vi "Read_I2C_Data.vi"(8 "Error_In":errorcluster, 11 "I2C_In":refnum<class "I2C.lvclass">) -> (0 "Error_Out":errorcluster, 2 "Convertor_Data":T1={"Vmin"=0.0, "Vmax"=1.0, "Input"="", "Off_Set (uS)"=0.0, "T_HD_STA (uS)"=0.0, "Sample_Per_Us"=0.0, "T_HD_DAT (uS)"=0.0, "T_SU_DAT (uS)"=0.0, "Frequency (kHz)"=0.0, "T_SU_STO"=0.0, "T_Off (uS)"=0.0, "T_On (uS)"=0.0, "T_BUF"=0.0, "Target_Address"=0, "Selected_Register_Address"=0, "Byte_Array"=[], "Target_Name"="", "Register_Name"=[], "Register_Address"=[], "Target_Type"=0, "Register_Data"=[]} {"Target_Type" items=["10 Bit Address", "7 Bit Address"]; "Selected_Register_Address" format="%x"; "Target_Address" format="%x"}, 3 "I2C_Out":refnum<class "I2C.lvclass">)   [LabVIEW 2021, in "I2C.lvclass"]
doc: "Used to Read the I2C data"
uses:
  I2C.lvclass
  Controls/I2C_Data.ctl
  Controls/Customized_Ring.ctl
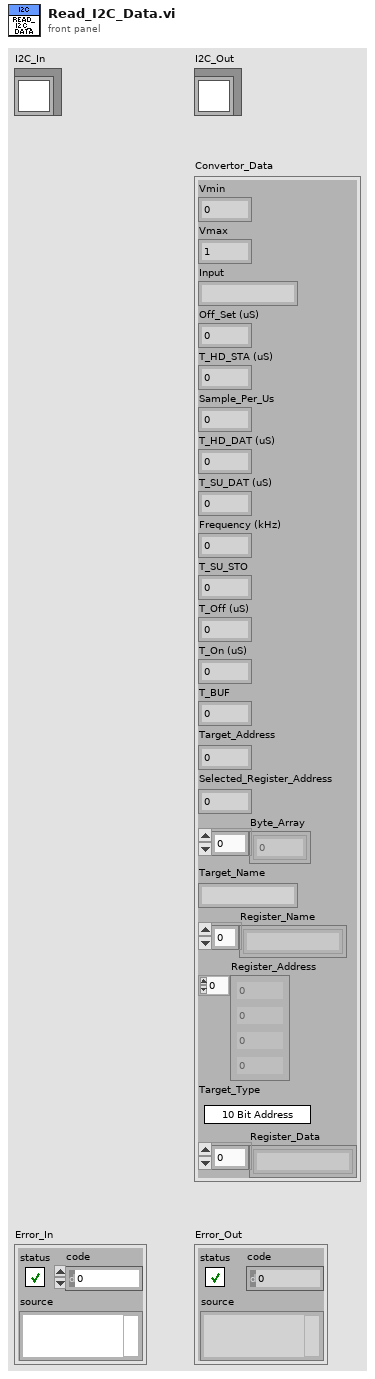
[diagram p1: front panel]
types:
  T1 = typedef "I2C_Data.ctl" = cluster{"Vmin":dbl, "Vmax":dbl, "Input":string, "Off_Set (uS)":dbl, "T_HD_STA (uS)":dbl, "Sample_Per_Us":dbl, "T_HD_DAT (uS)":dbl, "T_SU_DAT (uS)":dbl, "Frequency (kHz)":dbl, "T_SU_STO":dbl, "T_Off (uS)":dbl, "T_On (uS)":dbl, "T_BUF":dbl, "Target_Address":u16, "Selected_Register_Address":u8, "Byte_Array":u8[], "Target_Name":string, "Register_Name":string[], "Register_Address":u8[], "Target_Type":T2, "Register_Data":string[]}
  T2 = typedef "Customized_Ring.ctl" = u16
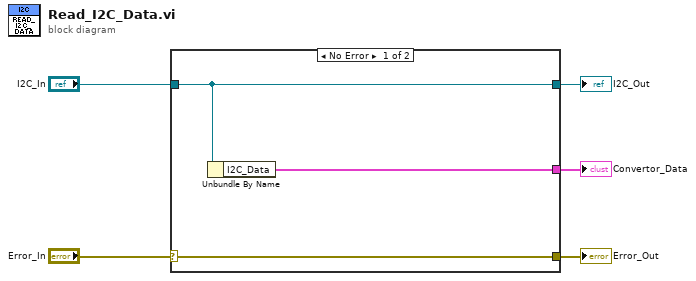
[diagram p0: block diagram]
diagram:
  n1 = case shown="No Error" "Error_In" {
    selector: "Error_In" -> [w8 w9]
    tunnel: [w8 w9] -> w4
    tunnel: [w7 w10] -> w2
    tunnel: "I2C_In" -> [w7 w10]
    tunnel: [w6 _] -> w1
    frame No Error {
      n2 = Unbundle By Name(w7) -> ("I2C_Data"=w6:T1)
    }
    frame Error {
    }
  }
  "Error_Out" <- w4
  "I2C_Out" <- w2
  "Convertor_Data" <- w1
